vi "BracePLUS_Main.vi"() -> ()   [LabVIEW 2018]
panel:
  in  "Tab Control":enum32{"Main", "Setup", "Files", "Tools"}(tab)
  out "Rep":i32
  in  "Participant Code":string
  out "Time":string
  in  "Filename":string
  in  "Quit Button":bool
  in  "Log Data Button":bool
  in  "Add Pcode":bool
  out "Participant ID":string
  in  "VISA resource name":refnum<visa-resource-name>="COM3"
  in  "Serial Settings":T1={"baud rate"=115200, "data bits"=8, "parity"=enum."None", "stop bits"=10, "flow control"=0} {"flow control" items=["None"=0, "XON/XOFF"=1, "RTS/CTS"=2, "DTR/DSR"=4]; "stop bits" items=["1.0"=10, "1.5"=15, "2.0"=20]; "data bits" min=5 max=8 step=1; "baud rate" items=["75"=75, "110"=110, "134"=134, "150"=150, "300"=300, "600"=600, "1200"=1200, "1800"=1800, "2400"=2400, "4800"=4800, "7200"=7200, "9600"=9600, "14400"=14400, "19200"=19200, "28800"=28800, "38400"=38400, "56000"=56000, "57600"=57600, "115200"=115200, "128000"=128000, "230400"=230400]}
  out "Data Path":path
  out "filenames":string[](array[string])
  in  "Retrieve Data Button":bool
  in  "View Saved Data":bool
  in  "Stream Button":bool
  # "Brace+"
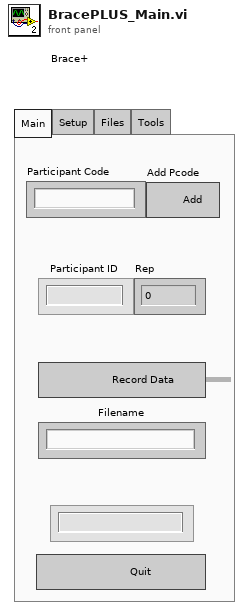
[diagram p1: front panel]
types:
  T1 = cluster{"baud rate":u32, "data bits":u16, "parity":enum16{"None", "Odd", "Even", "Mark", "Space"}, "stop bits":u16, "flow control":u16}
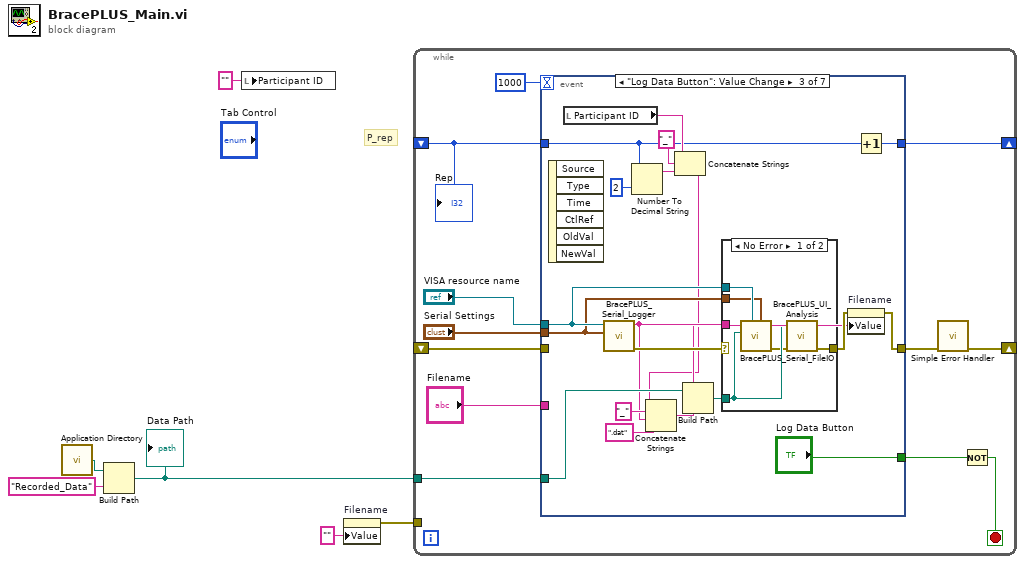
[diagram p0: block diagram]
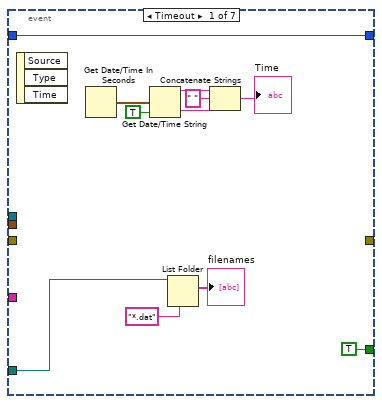
[diagram p2: hidden frame]
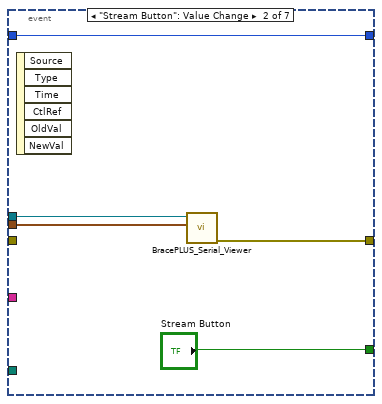
[diagram p3: hidden frame]
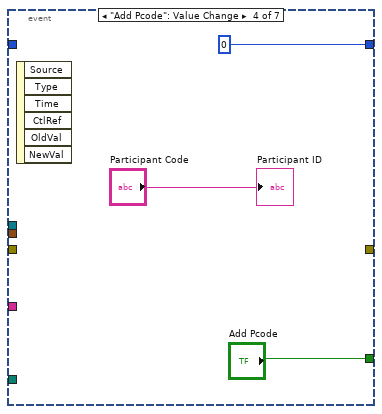
[diagram p5: hidden frame]
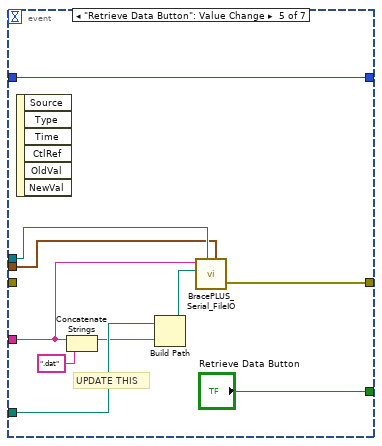
[diagram p6: hidden frame]
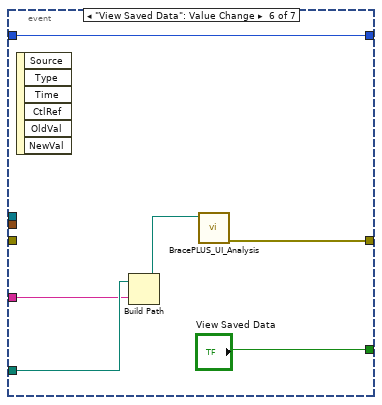
[diagram p7: hidden frame]
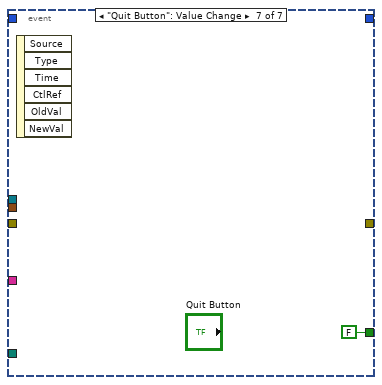
[diagram p8: hidden frame]
diagram:
  # "P_rep"
  n1 = call <vilib>:"Application Directory.vi"() -> ("Application Directory"=w4:path)
  n2 = Build Path(base path=w4, name or relative path="Recorded_Data" ("string")) -> (appended path=w2:path)
  "Data Path" <- w2
  n3 = local write "Participant ID"("" ("Participant ID")) -> ()
  n4 = property on="Filename" class="Str"("Value"="" ("Filename")) -> (error out=w3:errorcluster)  [unwired: 2 in, 1 out]
  n5 = while {
    shift-right: [w10] -> _
    shift-left: _ -> [w13]
    tunnel: w2 -> [w12]
    tunnel: w3 -> [_]
    shift-right: [w8] -> _
    shift-left: _ -> [w7]
    stop <- w17 stop-if-true
    n6 = event shown="[2] \"Log Data Button\": Value Change" {
      selector: _ -> [_ _ _ _ _ _ _]
      dyn-events: _ -> [_ _ _ _ _ _ _]
      timeout: 1000 -> [_ _ _ _ _ _ _]
      tunnel: [TRUE ("Stream Button") "Stream Button" "Log Data Button" "Add Pcode" "Retrieve Data Button" "View Saved Data" FALSE ("Stream Button")] -> w18
      tunnel: "VISA resource name" -> [_ w33 w49 _ w66 _ _]
      tunnel: "Serial Settings" -> [_ w32 w48 _ w65 _ _]
      tunnel: [_ w31 w53 _ w67 w76 _] -> w11
      tunnel: "Filename" -> [_ _ _ _ w70 w75 _]
      tunnel: w13 -> [_ _ _ _ _ _ _]
      tunnel: w12 -> [w27 _ w51 _ w71 w78 _]
      tunnel: w7 -> [w19 w30 w35 _ w64 w74 _]
      tunnel: [w19 w30 w36 0 w64 w74 _] -> w8
      event Timeout {
        n7 = event-data() -> ()  [unwired: 1 in, 3 out]
        n8 = Get Date/Time In Seconds() -> (seconds since 1Jan1904=w26:timestamp)
        n9 = Get Date/Time String(seconds (now)=w26, want seconds? (F)=TRUE) -> (date string=w22:string, time string=w23:string)  [unwired: 1 in]
        n10 = List Folder(path=w27, pattern="*.dat") -> (filenames=→"filenames":string[])  [unwired: 2 in, 3 out]
        n11 = Concatenate Strings(w22, " " ("string"), w23) -> (→"Time":string)
      }
      event "Stream Button": Value Change {
        n12 = event-data() -> ()  [unwired: 1 in, 6 out]
        n13 = call "BracePLUS_Serial_Viewer.vi"("Serial Settings"=w32, "VISA resource name"=w33) -> ("error out"=w31:errorcluster)  [unwired: 9 in]
      }
      event "Log Data Button": Value Change {
        n14 = event-data() -> ()  [unwired: 1 in, 6 out]
        n15 = local read "Participant ID"() -> (w42:string)
        n16 = call "BracePLUS_Serial_Logger.vi"("Serial Settings"=w48, "VISA resource name"=w49) -> ("error out"=w50:errorcluster, "Filename"=w44:string)  [unwired: 8 in]
        n17 = Number To Decimal String(number=w35, width (-)=i16 2) -> (decimal integer string=w39:string)
        n18 = Concatenate Strings(w42, "_" ("Filename"), w39) -> (w38:string)
        n19 = Concatenate Strings(w38, "_" ("Filename"), w44, ".dat" ("Filename")) -> (w41:string)
        n20 = Build Path(base path=w51, name or relative path=w41) -> (appended path=w47:path)
        n21 = case shown="No Error" w50 {
          selector: w50 -> [_ w60]
          tunnel: w49 -> [w59 _]
          tunnel: w48 -> [w58 _]
          tunnel: w44 -> [w57 _]
          tunnel: w47 -> [w56 _]
          tunnel: [w54 w60] -> w46
          frame No Error {
            n22 = call "BracePLUS_Serial_FileIO.vi"("Serial Settings"=w58, "VISA resource name"=w59, "Filename to Save to..."=w56, "Remote Filename"=w57) -> ("error out"=w55:errorcluster)  [unwired: 6 in, 1 out]
            n23 = call "BracePLUS_UI_Analysis.vi"("error in"=w55, "Path"=w56) -> ("error out"=w54:errorcluster)  [unwired: 9 in]
          }
          frame Error {
          }
        }
        n24 = property on="Filename" class="Str"(error in=w46, "Value"=w41) -> (error out=w53:errorcluster)  [unwired: 1 in, 1 out]
        n25 = Increment(x=w35) -> (x+1=w36:i32)
      }
      event "Add Pcode": Value Change {
        n26 = event-data() -> ()  [unwired: 1 in, 6 out]
        "Participant ID" <- "Participant Code"
      }
      event "Retrieve Data Button": Value Change {
        # "UPDATE THIS"
        n27 = event-data() -> ()  [unwired: 1 in, 6 out]
        n28 = Concatenate Strings(w70, ".dat" ("Filename")) -> (w69:string)
        n29 = Build Path(base path=w71, name or relative path=w69) -> (appended path=w72:path)
        n30 = call "BracePLUS_Serial_FileIO.vi"("Serial Settings"=w65, "VISA resource name"=w66, "Filename to Save to..."=w72, "Remote Filename"=w70) -> ("error out"=w67:errorcluster)  [unwired: 6 in, 1 out]
      }
      event "View Saved Data": Value Change {
        n31 = event-data() -> ()  [unwired: 1 in, 6 out]
        n32 = Build Path(base path=w78, name or relative path=w75) -> (appended path=w77:path)
        n33 = call "BracePLUS_UI_Analysis.vi"("Path"=w77) -> ("error out"=w76:errorcluster)  [unwired: 10 in]
      }
      event "Quit Button": Value Change {
        n34 = event-data() -> ()  [unwired: 1 in, 6 out]
      }
    }
    n35 = call <vilib>:"Simple Error Handler.vi"("error in (no error)"=w11) -> ("error out"=w10:errorcluster)  [unwired: 4 in, 4 out]
    n36 = Not(x=w18) -> (.not. x?=w17:bool)
    "Rep" <- w7
  }
